vi "Analog Read - TCP Connection.vi"() -> ()   [LabVIEW 2011, in "LVH-LINX.lvlib"]
doc: "Read one or more analog values from a LINX device using the LINX TCP interface."
uses:
  vi.lib/LabVIEW Hacker/LINX/LVH-LINX.lvlib
  vi.lib/LabVIEW Hacker/LINX/Private/Device/Type Defs/TCP Config.ctl
  vi.lib/LabVIEW Hacker/LINX/Private/Device/Device.lvlib
panel:
  in  "TCP Configuration":T1
  in  "Stop Button":bool
  out "Analog Data":T2(graph)
  in  "AI Channel(s)":u8[](array[numeric])=[0, 1, 2]
  # "Analog Values"
  # "LINX Device Settings"
  # "Analog Read Example (TCP Interface)\n\nThis example demonstrates how to read analog input values from a LINX device connected to the host computer via Serial / USB.\n\nInstructions\n1. Enter the IP Addres and Port associated with the LINX Device.\n2. Select the Analog Channel(s) to read.\n3. Click the Run Arrow."
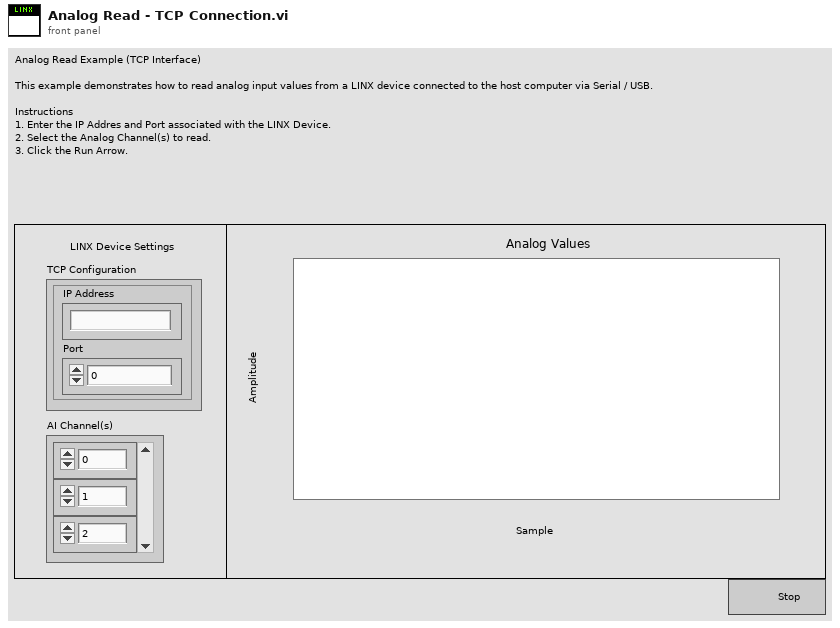
[diagram p1: front panel]
types:
  T1 = typedef "LVH-LINX.lvlib/Device.lvlib/TCP Config.ctl" = cluster{"IP Address":string, "Port":u16}
  T2 = cluster{"Voltages[0]":dbl, "Voltages[1]":dbl, "Voltages[2]":dbl, "Voltages[3]":dbl, "Voltages[4]":dbl, "Voltages[5]":dbl, "Voltages[6]":dbl, "Voltages[7]":dbl, "Voltages[8]":dbl}
  T3 = typedef "LVH-LINX.lvlib/LINX Ref.ctl" = cluster{"Platform":T4, "Interface":T5, "LINX Device Config":T6}
  T4 = typedef "LVH-LINX.lvlib/Platform.ctl" = enum16{"LINX", "myRIO"}
  T5 = typedef "LVH-LINX.lvlib/Interface.ctl" = enum16{"Serial", "TCP"}
  T6 = typedef "LVH-LINX.lvlib/Device.lvlib/LINX Device Config.ctl" = cluster{"Interface":T5, "COM Port":refnum<visa-resource-name>, "TCP Configuration":T1, "Device Family":T7, "Device ID":u8, "Device Name":string, "TCP Ref":refnum<k5>}
  T7 = typedef "LVH-LINX.lvlib/Device Family.ctl" = enum8{"National Instruments", "Digilent", "Arduino"}
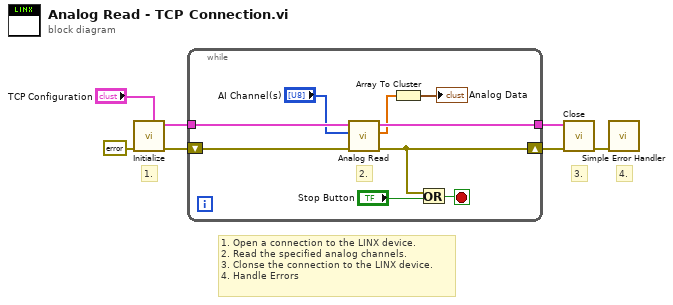
[diagram p0: block diagram]
diagram:
  # "1. Open a connection to the LINX device.\n2. Read the specified analog channels.\n3. Clonse the connection to the LINX device.\n4. Handle Errors"
  # "4."
  # "3."
  # "1."
  n1 = call "Initialize.vi"("TCP Configuration"="TCP Configuration", "Error In"=errorcluster {"status"=FALSE, "code"=0, "source"=""}) -> ("Error Out"=w6:errorcluster, "LINX Ref"=w7:T3)  [unwired: 8 in]
  n2 = while {
    tunnel: w7 -> [w16]
    tunnel: [w14] -> w5
    shift-right: [w10] -> w4
    shift-left: w6 -> [w15]
    stop <- w12 stop-if-true
    # "2."
    n3 = call "Analog Read.vi"("Error In"=w15, "AI Channel(s)"="AI Channel(s)", "LINX Resource"=w16) -> ("Error Out"=w10:errorcluster, "Voltages"=w9:dbl[], "LINX Resource"=w14:T3)  [unwired: 6 in]
    n4 = Array To Cluster(array=w9) -> (cluster=→"Analog Data":T2)
    n5 = Or(x=w10, y="Stop Button") -> (x .or. y?=w12:bool)
  }
  n6 = call "Close.vi"("Error In"=w4, "LINX Resource"=w5) -> ("Error Out"=w3:errorcluster)  [unwired: 8 in, 1 out]
  n7 = call <vilib>:"Simple Error Handler.vi"("error in (no error)"=w3) -> ()  [unwired: 4 in, 5 out]
